vi "Parse.vi"(8 "Error In":errorcluster, 11 "object in":refnum<class "2022_6.lvclass">) -> (0 "Error Out":errorcluster, 3 "object out":refnum<class "2022_6.lvclass">)   [LabVIEW 2020, in "2022_6.lvclass"]
uses:
  2022_6.lvclass
  2022_6.lvclass/2022_6.ctl
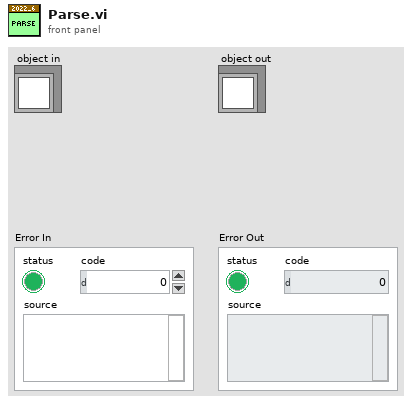
[diagram p1: front panel]
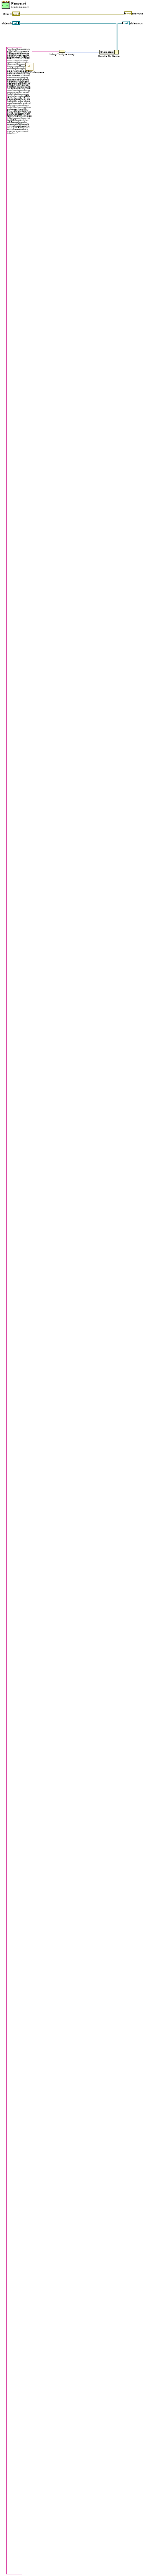
[diagram p0: block diagram]
diagram:
  n1 = call <vilib>:"Trim Whitespace.vi"("string"="mnlnvlljqqccznnjtjljbllrtllwwpmmhjjbbzppnndmmsppdqqwvvstvssgmsggmlmttnvvfbbdsssnzzbssjrsjjpmpvmmcjjwsssndsslwsswtwnwrrslshhvzzsppffmpfmmfvfpfpsssqpqzpqqcjcjnjcnnzbzjzpzbpbnbwbcctvvhgvgsvvpwwvjjvqjjjdqqrmrmqmsqszqsqpsqslsddhbhcbhbchcvvjvjcjnccdbcdcrddldblbffhvffpvpzpvvmvfmmwhwqhqvhqhmmpdmmlbmbgmbbrqqpmqqcvcmvvcncllptltvtdtbbqzzcggjgsjjvjsvvgmgffqhqqgpptspsffvdvbbhqhzzllvvjbvvbpppggfpgptgtvvzdvdzdgzgccmmphpmhppldlnlpnnhghhrrgwrwssnllmpllbvbvqvtvhtvvmnvvpgvgfvggtztpthhcfhfqfhhnhtnhhljhjppqjjffgjggrwrjjhphzhtztggwswnwzzvbzzmmtrtqtjqttwlwmmmmnddmnddwvvcllgrgfgzznwnsswjjhwwspsbbvzzqvzvbvcvmmtltnlnfn..." ("PuzzleInput")) -> ("trimmed string"=w2:string)  [unwired: 1 in]
  n2 = String To Byte Array(string=w2) -> (unsigned byte array=w1:u8[])
  n3 = Bundle By Name(cluster="object in", "Characters"=w1) -> (→"object out":refnum<class "2022_6.lvclass">)
  "Error Out" <- "Error In"
